vi "libssh2_knownhost_readfile - invalid known hosts collection - returns zero.vi"() -> ()   [LabVIEW 2017, in "unit_tests.lvlib"]
uses:
  unit_tests.lvlib
  libssh2/Host Key Database Refnum.ctl
  libssh2/libssh2_init_default.vi
  libssh2/libssh2_session_init_ex.vi
  libssh2/libssh2.lvlib
  <vilib>/PNR/Transparent Assertions/Transparent Assertions/Transparent Assertions.lvlib
panel:
  out "error out":errorcluster
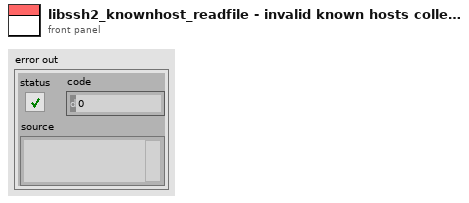
[diagram p1: front panel]
types:
  T1 = typedef "libssh2.lvlib/Session Refnum.ctl" = refnum<k1>
  T2 = typedef "libssh2.lvlib/Host Key Database Refnum.ctl" = refnum<k1>
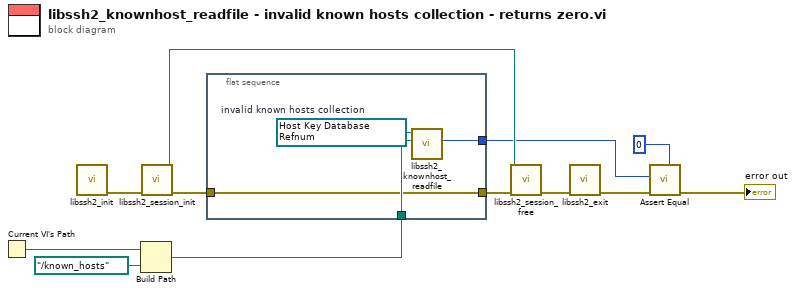
[diagram p0: block diagram]
diagram:
  n1 = Current VI's Path() -> (path=w5:path)
  n2 = call-poly "libssh2_init.vi"() -> ("error out"=w11:errorcluster)  [unwired: 11 in]
  n3 = Build Path(base path=w5, name or relative path=path "../known_hosts" ("filename")) -> (appended path=w3:path)
  n4 = call "libssh2_session_init.vi"("error in (no error)"=w11) -> ("error out"=w2:errorcluster, "session"=w8:T1)  [unwired: 9 in]
  n5 = flat-sequence {
    tunnel: [w16] -> w7
    tunnel: w3 -> [w14]
    tunnel: w2 -> [w13]
    tunnel: [w13] -> w1
    frame #0 {
      w15 = T2 refnum items=["host key database"]  # invalid known hosts collection
      n6 = call "libssh2_knownhost_readfile.vi"("filename"=w14, "host key database"=w15) -> ("hosts added"=w16:i32)  [unwired: 8 in, 1 out]
    }
  }
  n7 = call "libssh2_session_free.vi"("error in (no error)"=w1, "session"=w8) -> ("error out"=w10:errorcluster)  [unwired: 9 in]
  n8 = call "libssh2_exit.vi"("error in (no error)"=w10) -> ("error out"=w9:errorcluster)  [unwired: 10 in]
  n9 = call <vilib>:"Assert Equal.vi"("Expected"=0 ("hosts added"), "error in (no error)"=w9, "Actual"=w7) -> ("error out"=→"error out":errorcluster)  [unwired: 8 in]
